vi "膜版匹配.vi"(0 "Image In":T5, 1 "Image Dst":T5, 2 "Algorithm (Pattern Matching 1)":i32(ring)=2 items=["All", "Low Discrepancy Sampling", "Grayscale Value Pyramid", "Gradients Pyramid"], 3 "Parameters (Pattern Matching 1)":T4={"Number of Matches Requested"=1, "Minimum Match Score"=700.0, "Angle Ranges"=[{"Start Angle"=-45.0, "End Angle"=45.0}, {"Start Angle"=135.0, "End Angle"=225.0}]}, 4 "Advanced Options (Pattern Matching 1)":cluster{"Item":u16, "Value":dbl}[](array[cluster])=[{"Item"=102, "Value"=10.0}, {"Item"=106, "Value"=300.0}, {"Item"=107, "Value"=0.0}, {"Item"=108, "Value"=6.0}, {"Item"=109, "Value"=1.0}, {"Item"=114, "Value"=25.0}, {"Item"=111, "Value"=20.0}, {"Item"=112, "Value"=10.0}, {"Item"=113, "Value"=20.0}, {"Item"=103, "Value"=1.0}, {"Item"=104, "Value"=20.0}, {"Item"=105, "Value"=0.0}, {"Item"=100, "Value"=7.0}] {"Item" items=["LD Sampling - Minimum Constrast"=0, "LD Sampling - Enable Subpixel Accuracy"=1, "LD Sampling - Search Strategy"=2, "LD Sampling - Subpixel Iterations"=3, "LD Sampling - Subpixel Tolerance"=4, "LD Sampling - Initial Match List Length"=5, "LD Sampling - Match List Reduction Factor"=6, "LD Sampling - Initial Step Size"=7, "LD Sampling - Intermediate Angular Accuracy"=8, "-"=9, "Pyramid - Max Pyramid Level"=100, "Pyramid - Minimum Contrast"=102, "Pyramid - Enable Subpixel Accuracy"=103, "Pyramid - Subpixel Iterations"=104, "Pyramid - Subpixel Tolerance"=105, "Pyramid - Initial Match List Length"=106, "Pyramid - Match List Reduction Factor"=107, "Pyramid - Intermediate Angular Accuracy"=108, "Pyramid - Process Border Matches"=109, "Pyramid - Min Match Separation Distance"=111, "Pyramid - Min Match Separation Angle"=112, "Pyramid - Max Match Overlap"=113, "Pyramid - Max Cache in MB"=114, "Pyramid - Clear Cache"=115, "-"=116, "Enable Defect Map"=200]}, 5 "Template File Path (Pattern Matching 1)":path=path "D:/Inspect System/Source Code/Template Program/字符检测定位模板.png", 6 "ROI Descriptor (OCR/OCV 1)":T3={"Global Rectangle"=[161, 817, 841, 909], "Contours"=[{"ID"=enum."External", "Type"=12, "Coordinates"=[162, 818, 840, 908, 19]}]} {"Contours"."Type" items=["No Selection", "Point", "Line", "Rectangle", "Oval", "Polygon", "Freehand Region", "Annulus", "Unused2", "Unused3", "Broken Line", "Freehand Line", "Rotated Rectangle"]}, 7 "error in":errorcluster, 8 "File Path (OCR/OCV 1)":path=path "D:/Inspect System/Source Code/SubVIs/字符检测VI/字符模板数字.abc", 9 "Parameters (OCR/OCV 1)":T2={"Threshold Data"={"Method"=enum."Uniform", "Looking for"=1, "Color Mode"=0, "Kernel Size"={"Width"=32, "Height"=32}, "Ranges"=[{"Min"=1, "Max"=255}]}, "Reject Border"=FALSE, "Number Of Erosions"=0, "Size & Spacing"={"Segment Algorithm"=0, "Min Bounding Rect Width"=1, "Max Bounding Rect Width"=65, "Min Bounding Rect Height"=1, "Max Bounding Rect Height"=65536, "Min Character Size"=20, "Max Character Size"=65536, "Min Char Spacing"=1, "Max Horiz Element Spacing"=1, "Max Vert Element Spacing"=0, "Max Space Distance"=65536}, "Read Options"={"Read Strategy"=1, "Read Resolution"=2, "Scale Dependant"=FALSE, "Aspect Ratio"=400, "Acceptance Level"=700, "Substitution Character"="?", "MultiLine"=TRUE}, "Valid Characters"=[], "Use Text Pattern"=FALSE, "Orientation"=0, "# Lines Expected"=0, "Number of Blocks"=4} {"Threshold Data"."Looking for" items=["Light on Dark", "Dark on Light"]; "Threshold Data"."Color Mode" items=["RGB", "HSL", "HSV", "HSI"]; "Size & Spacing"."Segment Algorithm" items=["None", "Shortest Segment", "Legacy Auto Split"]; "Read Options"."Read Strategy" items=["Aggressive", "Conservative"]; "Read Options"."Read Resolution" items=["Low", "Medium", "High"]; "Valid Characters"."Pre-defined characters" items=["Any Character", "User-defined Characters", "Alphabetic", "Alphanumeric", "Uppercase Letters", "Lowercase Letters", "Decimal Digits", "Hexadecimal Digits", "Pattern", "Force Space"]; "Orientation" items=["Baseline inside", "Baseline outside"]}, 10 "Coordinate System Out":T1 {"Measurement System"."Axis Reference" items=["Direct", "Indirect"]; "Measurement System"."Angle (deg)" format="%.2f"; "Measurement System"."Origin"."Y" format="%.2f"; "Measurement System"."Origin"."X" format="%.2f"; "Reference System"."Axis Reference" items=["Direct", "Indirect"]; "Reference System"."Angle (deg)" format="%.2f"; "Reference System"."Origin"."Y" format="%.2f"; "Reference System"."Origin"."X" format="%.2f"}) -> (20 "Image Out":T5, 21 "Matches (Pattern Matching 1)":T8(array[cluster]) {"Bounding Box"."y" format="%.2f"; "Bounding Box"."x" format="%.2f"; "Position"."y" format="%.2f"; "Position"."x" format="%.2f"; "Score" format="%.2f"; "Scale" format="%.2f"; "Angle" format="%.2f"}, 22 "String (OCR/OCV 1)":string, 23 "OCR Session (OCR/OCV 1)":T6, 24 "Number of Matches (Pattern Matching 1)":i32, 25 "Coordinate System Out (Set Coordinate System 1)":T7 {"Measurement System"."Axis Reference" items=["Direct", "Indirect"]; "Measurement System"."Angle (deg)" format="%.2f"; "Measurement System"."Origin"."Y" format="%.2f"; "Measurement System"."Origin"."X" format="%.2f"; "Reference System"."Axis Reference" items=["Direct", "Indirect"]; "Reference System"."Angle (deg)" format="%.2f"; "Reference System"."Origin"."Y" format="%.2f"; "Reference System"."Origin"."X" format="%.2f"}, 27 "error out":errorcluster)   [LabVIEW 2017]
doc: "Creates, edits, and runs vision algorithms using NI Vision Assistant.\n\nWhen you place this Express VI on the block diagram, NI Vision Assistant launches. Create an algorithm using the Vision Assistant processing functions. After you create an algorithm, you can select the controls and indicators that you want to be able to programmatically set in LabVIEW. Double-click the Vision Assistant Express VI to edit the algorithm."
uses:
  <vilib>/vision/Image Controls.llb/IMAQ Image.ctl
  <vilib>/vision/OCR.llb/IMAQ OCR Session.ctl
  <vilib>/vision/NI_Vision_Development_Module.lvlib
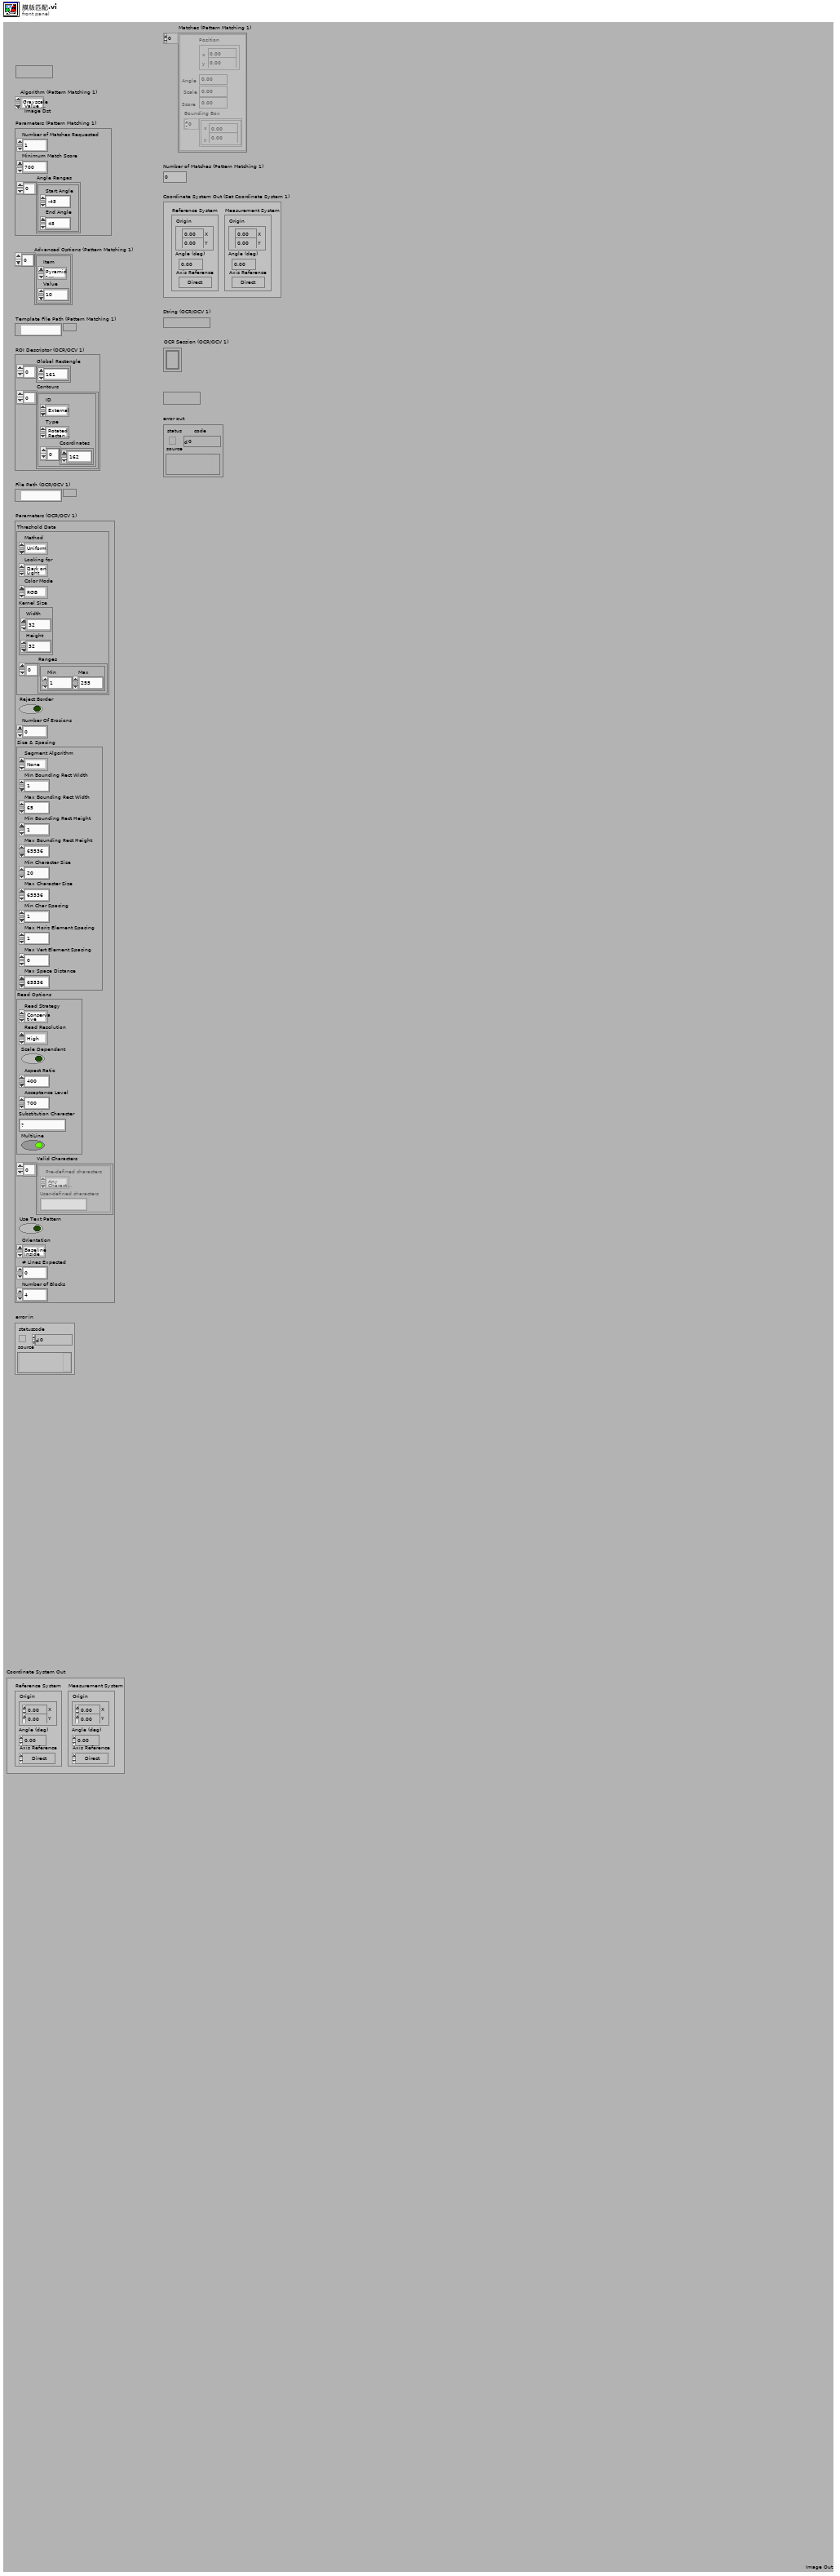
[diagram p1: front panel]
types:
  T1 = typedef "IMAQ Coordinate System" = cluster{"Reference System":cluster{"Origin":cluster{"X":sgl, "Y":sgl}, "Angle (deg)":sgl, "Axis Reference":u32}, "Measurement System":cluster{"Origin":cluster{"X":sgl, "Y":sgl}, "Angle (deg)":sgl, "Axis Reference":u32}}
  T2 = cluster{"Threshold Data":cluster{"Method":enum16{"Fixed Range", "Uniform", "Linear", "Non Linear", "Local", "Color"}, "Looking for":u32, "Color Mode":u32, "Kernel Size":cluster{"Width":i32, "Height":i32}, "Ranges":cluster{"Min":i32, "Max":i32}[]}, "Reject Border":bool, "Number Of Erosions":i32, "Size & Spacing":cluster{"Segment Algorithm":u16, "Min Bounding Rect Width":i32, "Max Bounding Rect Width":i32, "Min Bounding Rect Height":i32, "Max Bounding Rect Height":i32, "Min Character Size":i32, "Max Character Size":i32, "Min Char Spacing":i32, "Max Horiz Element Spacing":i32, "Max Vert Element Spacing":i32, "Max Space Distance":i32}, "Read Options":cluster{"Read Strategy":i32, "Read Resolution":i32, "Scale Dependant":bool, "Aspect Ratio":i32, "Acceptance Level":i32, "Substitution Character":string, "MultiLine":bool}, "Valid Characters":cluster{"Pre-defined characters":i32, "User-defined characters":string}[], "Use Text Pattern":bool, "Orientation":u32, "# Lines Expected":u32, "Number of Blocks":i32}
  T3 = cluster{"Global Rectangle":i32[], "Contours":cluster{"ID":enum32{"External", "Internal"}, "Type":u32, "Coordinates":i32[]}[]}
  T4 = cluster{"Number of Matches Requested":i32, "Minimum Match Score":sgl, "Angle Ranges":cluster{"Start Angle":sgl, "End Angle":sgl}[]}
  T5 = typedef "IMAQ Image.ctl" = refnum<image>
  T6 = typedef "IMAQ OCR Session.ctl" = refnum<k1>
  T7 = cluster{"Reference System":cluster{"Origin":cluster{"X":sgl, "Y":sgl}, "Angle (deg)":sgl, "Axis Reference":u32}, "Measurement System":cluster{"Origin":cluster{"X":sgl, "Y":sgl}, "Angle (deg)":sgl, "Axis Reference":u32}}
  T8 = cluster{"Position":cluster{"x":sgl, "y":sgl}, "Angle":sgl, "Scale":sgl, "Score":sgl, "Bounding Box":cluster{"x":sgl, "y":sgl}[]}[]
  T9 = typedef "Image Type" = u32
  T10 = cluster{"Origin":cluster{"X":sgl, "Y":sgl}, "Angle (deg)":sgl, "Axis Reference":u32}
  T11 = enum16{"Reset", "Update Coordinate System", "Get Coordinate System"}
  T12 = enum16{"Horizontal Motion", "Vertical Motion", "Horizontal and Vertical Motion", "Horizontal, Vertical and Angular Motion"}
  T13 = typedef "ROI Descriptor" = cluster{"Global Rectangle":i32[], "Contours":cluster{"ID":enum32{"External", "Internal"}, "Type":u32, "Coordinates":i32[]}[]}
  T14 = cluster{"Backup Image Name":string, "Coordinate System Out":T1}
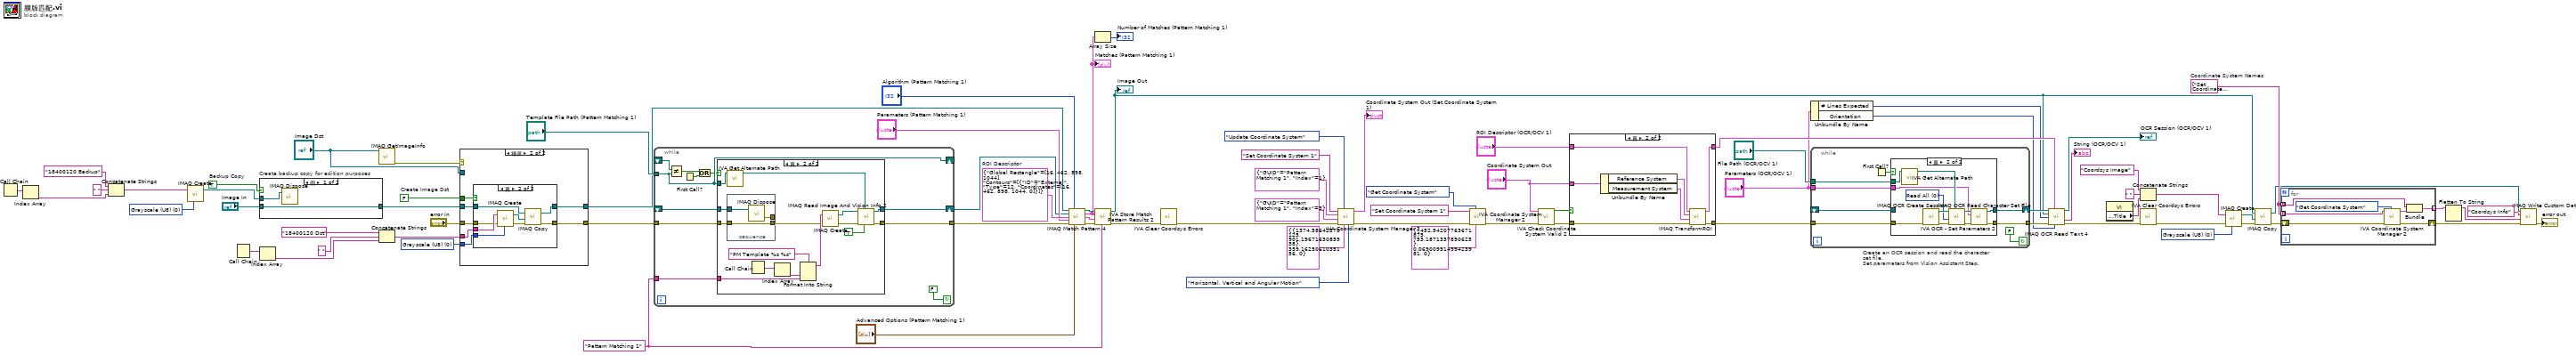
[diagram p0: block diagram]
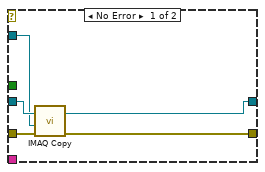
[diagram p5: hidden frame]
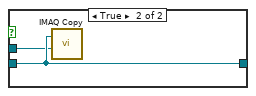
[diagram p7: hidden frame]
diagram:
  w5 = T9 0 items=["Grayscale (U8)", "Grayscale (I16)", "Grayscale (SGL)", "Complex (CSG)", "RGB (U32)", "HSL (U32)", "RGB (U64)", "Grayscale (U16)"] ("Image Type")
  w12 = string[] ["Set Coordinate System 1"]  # Coordinate System Names
  w52 = "Pattern Matching 1" ("Step Name")
  w55 = T3 {"Global Rectangle"=[16, 462, 898, 1044], "Contours"=[{"ID"=enum."External", "Type"=12, "Coordinates"=[16, 462, 898, 1044, 0]}]}  # ROI Descriptor
  w61 = T9 0 items=["Grayscale (U8)", "Grayscale (I16)", "Grayscale (SGL)", "Complex (CSG)", "RGB (U32)", "HSL (U32)", "RGB (U64)", "Grayscale (U16)"] ("Image Dst Type")
  w62 = T9 0 items=["Grayscale (U8)", "Grayscale (I16)", "Grayscale (SGL)", "Complex (CSG)", "RGB (U32)", "HSL (U32)", "RGB (U64)", "Grayscale (U16)"] ("Image Type")
  w81 = TRUE  # Backup Copy
  w74 = FALSE  # Create Image Dst
  n1 = Call Chain() -> (call chain=w68:string[])
  n2 = Index Array(array=w68) -> (element=w67:string)  [unwired: 1 in]
  n3 = Concatenate Strings("18400120 Backup" ("Backup Image Name"), " ", w67) -> (w64:string)
  n4 = call "IMAQ Create"("Image Name"=w64, "Image Type"=w62) -> ("New Image"=w63:T5)  [unwired: 2 in, 2 out]
  n5 = Call Chain() -> (call chain=w73:string[])
  n6 = case "Create backup copy for edition purposes" shown="假" w81 {
    tunnel: [w83 w85] -> w77
    tunnel: "Image In" -> [w83 w85]
    tunnel: w63 -> [w82 w84]
    frame False {
      n7 = call "IMAQ Dispose"("Image"=w82) -> ()  [unwired: 2 in, 4 out]
    }
    frame True {
      n8 = call "IMAQ Copy"("Image Dst"=w84, "Image Src"=w85) -> ()  [unwired: 1 in, 5 out]
    }
  }
  n9 = Index Array(array=w73) -> (element=w71:string)  [unwired: 1 in]
  n10 = call "IMAQ GetImageInfo"("Image"="Image Dst") -> ("error out"=w79:errorcluster)  [unwired: 1 in, 9 out]
  n11 = Concatenate Strings("18400120 Dst" ("Image Dst Name"), " ", w71) -> (w69:string)
  n12 = case "条件结构" shown="错误" w79 {
    tunnel: [w90 w94] -> w59
    tunnel: [w89 w93] -> w75
    tunnel: w77 -> [w88 w95]
    tunnel: "error in" -> [w87 w91]
    tunnel: "Image Dst" -> [w86 _]
    tunnel: w69 -> [_ w97]
    tunnel: w61 -> [_ w96]
    tunnel: w74 -> [_ w92]
    frame No Error {
      n13 = call "IMAQ Copy"("error in (no error)"=w87, "Image Dst"=w86, "Image Src"=w88) -> ("error out"=w89:errorcluster, "Image Dst Out"=w90:T5)  [unwired: 3 out]
    }
    frame Error {
      n14 = case "条件结构" shown="真" w92 {
        tunnel: w97 -> [_ w107]
        tunnel: w96 -> [_ w106]
        tunnel: w95 -> [w99 w104]
        tunnel: [w99 w103] -> w94
        tunnel: [w98 w102] -> w93
        tunnel: w91 -> [w98 w100]
        frame False {
        }
        frame True {
          n15 = call "IMAQ Create"("Image Name"=w107, "Image Type"=w106, "error in (no error)"=w100) -> ("New Image"=w105:T5, "error out"=w101:errorcluster)  [unwired: 1 in, 1 out]
          n16 = call "IMAQ Copy"("error in (no error)"=w101, "Image Dst"=w105, "Image Src"=w104) -> ("error out"=w102:errorcluster, "Image Dst Out"=w103:T5)  [unwired: 3 out]
        }
      }
    }
  }
  n17 = while {
    shift-right: [w118] -> w49
    shift-left: _ -> [w117]
    tunnel: [w115] -> w48
    tunnel: w75 -> [w114]
    tunnel: "Template File Path (Pattern Matching 1)" -> [w111]
    tunnel: w52 -> [w113]
    shift-right: [w111] -> _
    shift-left: _ -> [w112]
    stop <- FALSE continue-if-true
    n18 = Not Equal?(x=w112, y=w111) -> (x != y?=w109:bool)
    n19 = First Call?() -> (First Call?: T/F=w110:bool)
    n20 = Or(x=w109, y=w110) -> (x .or. y?=w108:bool)
    n21 = case "条件结构" shown="真" w108 {
      tunnel: [w120 w125] -> w118
      tunnel: w117 -> [w120 w129]
      tunnel: [w119 w126] -> w115
      tunnel: w114 -> [w119 w128]
      tunnel: w111 -> [_ w130]
      tunnel: w113 -> [_ w131]
      frame False {
      }
      frame True {
        n22 = call <vilib>:"IVA Get Alternate Path.vi"("Path In"=w130) -> ("Path Out"=w127:path)  [unwired: 10 out]
        n23 = stacked-sequence "层叠式顺序结构" {
          tunnel: w129 -> [w138]
          tunnel: w128 -> [w137]
          tunnel: [w137] -> w122
          tunnel: [w136] -> _
          frame #0 {
            n24 = call "IMAQ Dispose"("Image"=w138) -> ("error out"=w136:errorcluster)  [unwired: 2 in, 3 out]
          }
        }
        n25 = Call Chain() -> (call chain=w133:string[])
        n26 = Index Array(array=w133) -> (element=w132:string)  [unwired: 1 in]
        n27 = Format Into String(format string="PM Template %s %s" ("Image Name"), w132, w131) -> (resulting string=w135:string)  [unwired: 2 in, 1 out]
        n28 = call "IMAQ Create"("Image Name"=w135, "error in (no error)"=w122) -> ("New Image"=w124:T5, "error out"=w123:errorcluster)  [unwired: 2 in, 1 out]
        n29 = call "IMAQ Read Image And Vision Info 2"("Use File Path Image Type"=TRUE, "File Path"=w127, "error in (no error)"=w123, "Image"=w124) -> ("error out"=w126:errorcluster, "Image Out"=w125:T5)  [unwired: 5 in, 1 out]
      }
    }
  }
  n30 = call "IMAQ Match Pattern 4"("Image"=w59, "Algorithm"="Algorithm (Pattern Matching 1)", "Template Image"=w49, "ROI Descriptor"=w55, "Parameters"="Parameters (Pattern Matching 1)", "error in (no error)"=w48, "Advanced Options"="Advanced Options (Pattern Matching 1)") -> ("Image (duplicate)"=w57:T5, "Matches (pixel)"=w51:T8, "Matches (real-world)"=w50:T8, "error out"=w58:errorcluster)  [unwired: 4 in, 1 out]
  "Matches (Pattern Matching 1)" <- w51
  n31 = Array Size(array=w51) -> (size(s)=→"Number of Matches (Pattern Matching 1)":i32)
  n32 = call <vilib>:"IVA Store Match Pattern Results 2.vi"("Step Name"=w52, "error in (no error)"=w58, "Matches (real-world)"=w50, "Matches (pixel)"=w51, "Image in"=w57) -> ("error out"=w47:errorcluster, "Image dup"=w2:T5)  [unwired: 1 in, 4 out]
  "Image Out" <- w2
  n33 = call <vilib>:"IVA Clear Coordsys Errors.vi"("error in (no error)"=w47) -> ("error out"=w46:errorcluster)  [unwired: 10 in]
  n34 = call <vilib>:"IVA Coordinate System Manager 2.vi"("Mode"=T12."Horizontal, Vertical and Angular Motion", "Reference System"=T10 {"Origin"={"X"=1374.5864, "Y"=901.1967}, "Angle (deg)"=359.1625, "Axis Reference"=0}, "Function"=T11."Update Coordinate System", "error in (no error)"=w46, "Angle ID"=cluster{"GUID":string, "Index":i32} {"GUID"="Pattern Matching 1", "Index"=3}, "Origin ID"=cluster{"GUID":string, "Index":i32} {"GUID"="Pattern Matching 1", "Index"=1}, "Coordinate System Name"="Set Coordinate System 1") -> ("error out"=w38:errorcluster, "Coordinate System Out"=→"Coordinate System Out (Set Coordinate System 1)":T1)  [unwired: 3 out]
  n35 = call <vilib>:"IVA Coordinate System Manager 2.vi"("Reference System"=T10 {"Origin"={"X"=452.94208, "Y"=753.18713}, "Angle (deg)"=0.069009915, "Axis Reference"=0}, "Function"=T11."Get Coordinate System", "error in (no error)"=w38, "Coordinate System Name"="Set Coordinate System 1") -> ("error out"=w34:errorcluster)  [unwired: 3 in, 4 out]
  n36 = call <vilib>:"IVA Check Coordinate System Valid 2.vi"("error in (no error)"=w34, "Coordinate System"="Coordinate System Out") -> ("error out"=w29:errorcluster, "Valid?"=w30:bool)  [unwired: 8 out]
  n37 = case "条件结构" shown="真" w30 {
    tunnel: "ROI Descriptor (OCR/OCV 1)" -> [w140 w147]
    tunnel: [w140 w144] -> w26
    tunnel: [w139 w143] -> w31
    tunnel: "Coordinate System Out" -> [_ w142]
    tunnel: w29 -> [w139 w141]
    frame False {
    }
    frame True {
      n38 = Unbundle By Name(w142) -> ("Reference System"=w146:T10, "Measurement System"=w145:T10)
      n39 = call "IMAQ TransformROI"("error in (no error)"=w141, "New Reference"=w145, "Base Reference"=w146, "ROI Descriptor"=w147) -> ("error out"=w143:errorcluster, "ROI Descriptor out"=w144:T13)  [unwired: 6 out]
    }
  }
  n40 = Unbundle By Name("Parameters (OCR/OCV 1)") -> ("# Lines Expected"=w20:u32, "Orientation"=w21:u32)
  n41 = while "Create an OCR session and read the character set file.\nSet paramaters from Vision Assistant Step." {
    shift-right: [w152] -> w22
    shift-left: _ -> [w151]
    tunnel: w31 -> [w154]
    tunnel: "Parameters (OCR/OCV 1)" -> [w150]
    tunnel: "File Path (OCR/OCV 1)" -> [w149]
    tunnel: [w148] -> w23
    stop <- FALSE continue-if-true
    n42 = First Call?() -> (First Call?: T/F=w153:bool)
    n43 = case "条件结构" shown="真" w153 {
      tunnel: w149 -> [_ w161]
      tunnel: w154 -> [w156 w165]
      tunnel: [w157 w163] -> w152
      tunnel: [w156 w162] -> w148
      tunnel: w150 -> [_ w158]
      tunnel: w151 -> [w157 _]
      frame False {
      }
      frame True {
        w166 = 0 items=["Read All", "Read Character Set Only", "Read Properties Only"] ("Read Options")
        n44 = call <vilib>:"IVA Get Alternate Path.vi"("Path In"=w161) -> ("Path Out"=w160:path)  [unwired: 10 out]
        n45 = call "IMAQ OCR Create Session"("error in (no error)"=w165) -> ("error out"=w167:errorcluster, "IMAQ OCR Session"=w168:T6)  [unwired: 9 out]
        n46 = call "IMAQ OCR Read Character Set File"("File Path"=w160, "error in (no error)"=w167, "Read Options"=w166, "IMAQ OCR Session"=w168) -> ("error out"=w164:errorcluster, "IMAQ OCR Session (dup)"=w159:T6)  [unwired: 1 in, 5 out]
        n47 = call <vilib>:"IVA OCR - Set Parameters 2.vi"("error in (no error)"=w164, "Parameters"=w158, "IMAQ OCR Session"=w159) -> ("error out"=w162:errorcluster, "IMAQ OCR Session Out"=w163:T6)  [unwired: 7 in]
      }
    }
  }
  n48 = call "IMAQ OCR Read Text 4"("IMAQ OCR Session"=w22, "ROI Descriptor"=w26, "Image"=w2, "Number of Lines Requested"=w20, "error in (no error)"=w23, "Orientation"=w21) -> ("IMAQ OCR Session (dup)"=→"OCR Session (OCR/OCV 1)":T6, "Read String"=→"String (OCR/OCV 1)":string, "error out"=w19:errorcluster)  [unwired: 7 out]
  n49 = property class="VI"() -> ("Front Panel Window:Title"=w6:string)  [unwired: 2 in, 2 out]
  n50 = Concatenate Strings("Coordsys Image" ("Processed Image Name"), " ", w6) -> (w15:string)
  n51 = call <vilib>:"IVA Clear Coordsys Errors.vi"("error in (no error)"=w19) -> ("error out"=w18:errorcluster)  [unwired: 10 in]
  n52 = call "IMAQ Create"("Image Name"=w15, "Image Type"=w5, "error in (no error)"=w18) -> ("New Image"=w13:T5, "error out"=w14:errorcluster)  [unwired: 1 in, 1 out]
  n53 = call "IMAQ Copy"("error in (no error)"=w14, "Image Dst"=w13, "Image Src"=w2) -> ("error out"=w4:errorcluster, "Image Dst Out"=w11:T5)  [unwired: 3 out]
  n54 = for "For循环" {
    tunnel: w12 -> [w174] mode=indexing
    tunnel: w12 -> [w172] mode=indexing
    tunnel: [w171] -> w10 mode=indexing
    shift-right: [w169] -> w3
    shift-left: w4 -> [w170]
    n55 = call <vilib>:"IVA Coordinate System Manager 2.vi"("Function"=T11."Get Coordinate System", "error in (no error)"=w170, "Coordinate System Name"=w174) -> ("error out"=w169:errorcluster, "Coordinate System Out"=w173:T1)  [unwired: 4 in, 3 out]
    n56 = Bundle("Backup Image Name"=w172, "Coordinate System Out"=w173) -> (w171:T14)  [unwired: 1 out]
  }
  n57 = Flatten To String(anything=w10) -> (data string=w9:string)  [unwired: 1 in, 4 out]
  n58 = call "IMAQ Write Custom Data"("error in (no error)"=w3, "Custom Data In"=w9, "Key"="Coordsys Info", "Image"=w11) -> ("error out"=→"error out":errorcluster)  [unwired: 7 out]
